vi "closeInterface.vi"() -> ()   [LabVIEW 2018, in "MotorControllerClass.lvclass"]
uses:
  BMS/MotorControllerClass.lvclass
  <vilib>/CANopenLib/CANOPEN.llb/CANopen Interface Close.vi
panel:
  in  "MotorControllerClass in":refnum<class "MotorControllerClass.lvclass">
  out "MotorControllerClass in":refnum<class "MotorControllerClass.lvclass">
  in  "interface object in":refnum<k20>
  out "error out":errorcluster
  in  "error in (no error)":errorcluster
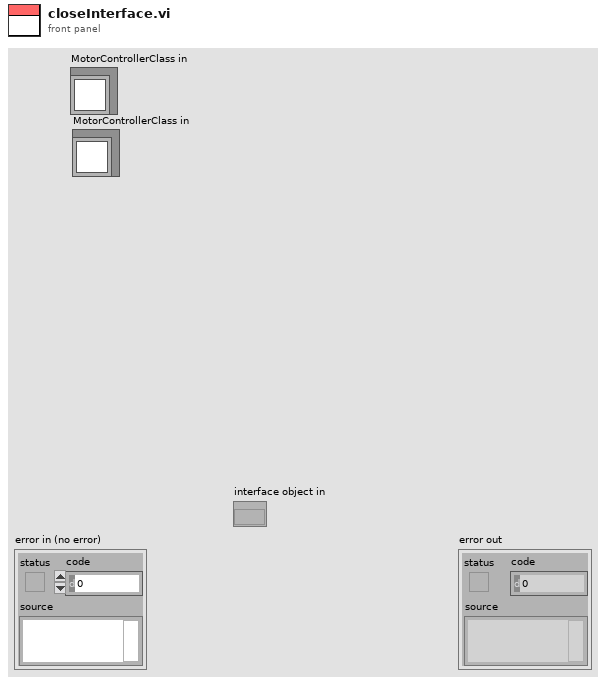
[diagram p1: front panel]
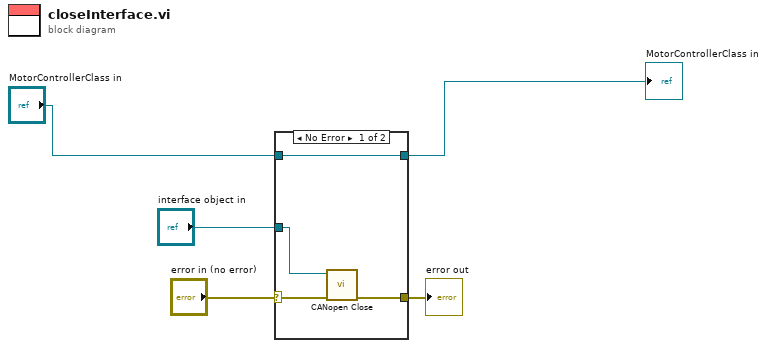
[diagram p0: block diagram]
diagram:
  n1 = case shown="No Error" "error in (no error)" {
    selector: "error in (no error)" -> [w8 w11]
    tunnel: [w7 w11] -> w4
    tunnel: [w9 w10] -> w2
    tunnel: "MotorControllerClass in" -> [w9 w10]
    tunnel: "interface object in" -> [w6 _]
    frame No Error {
      n2 = call-poly <vilib>:"CANopen Close.vi"("error in (no error)"=w8, "interface object in"=w6) -> ("error out"=w7:errorcluster)  [unwired: 9 in]
    }
    frame Error {
    }
  }
  "error out" <- w4
  "MotorControllerClass in" <- w2
